vi "DetectCollisionImproved.vi"(0 "ball":dbl[](array[numeric]), 3 "ignoreBall?":bool, 4 "Goal":dbl[](array[numeric]), 5 "our_robots":T1[](array[typedef]), 6 "Initial State":dbl[](array[numeric]), 7 "enemy_robots":T1[](array[typedef]), 8 "Is not first robot?":bool, 9 "element being analyzed":dbl[](array[numeric]), 10 "element already in path":dbl[](array[numeric]), 11 "Robot in":T1={"id"=0, "function"=enum."Attacker", "x"=0.0, "y"=0.0, "orientation"=0.0, "v_tangent"=0.0, "v_normal"=0.0, "v_ang"=0.0, "kick_x"=0.0, "kick_z"=0.0, "dribble"=FALSE, "Timestamp"=timestamp(0 s since 1904-01-01), "estimatives"={"est_v_tangent"=0.0, "est_v_normal"=0.0, "est_vx"=0.0, "est_vy"=0.0, "Pos Robot Est"=[]}, "dest_x_kick"=0.0, "dest_y_kick"=0.0, "Gap Coord"=[], "States"=enum."Pass", "Path "=[], "Path  Smooth"=[], "Dest"=[], "vx_desired"=0.0, "vy_desired"=0.0}) -> (2 "Is there colision?":bool)   [LabVIEW 2018]
uses:
  Vision_class/Old vision/Controls/AI Robot.ctl
  Vision_class/Old vision/Controls/Functions Enum.ctl
  Vision_class/Old vision/Controls/AttackerStates.ctl
  Vision_class/Old vision/Controls/PathDests.ctl
  Vision_class/Old vision/Controls/PathDest.ctl
  <vilib>/Analysis/_algsub.llb/Real Vector Norm.vi
  <vilib>/Analysis/baseanly.llb/Real Dot Product.vi
  <vilib>/Analysis/NI_AALBase.lvlib
  <vilib>/Analysis/NI_AALPro.lvlib
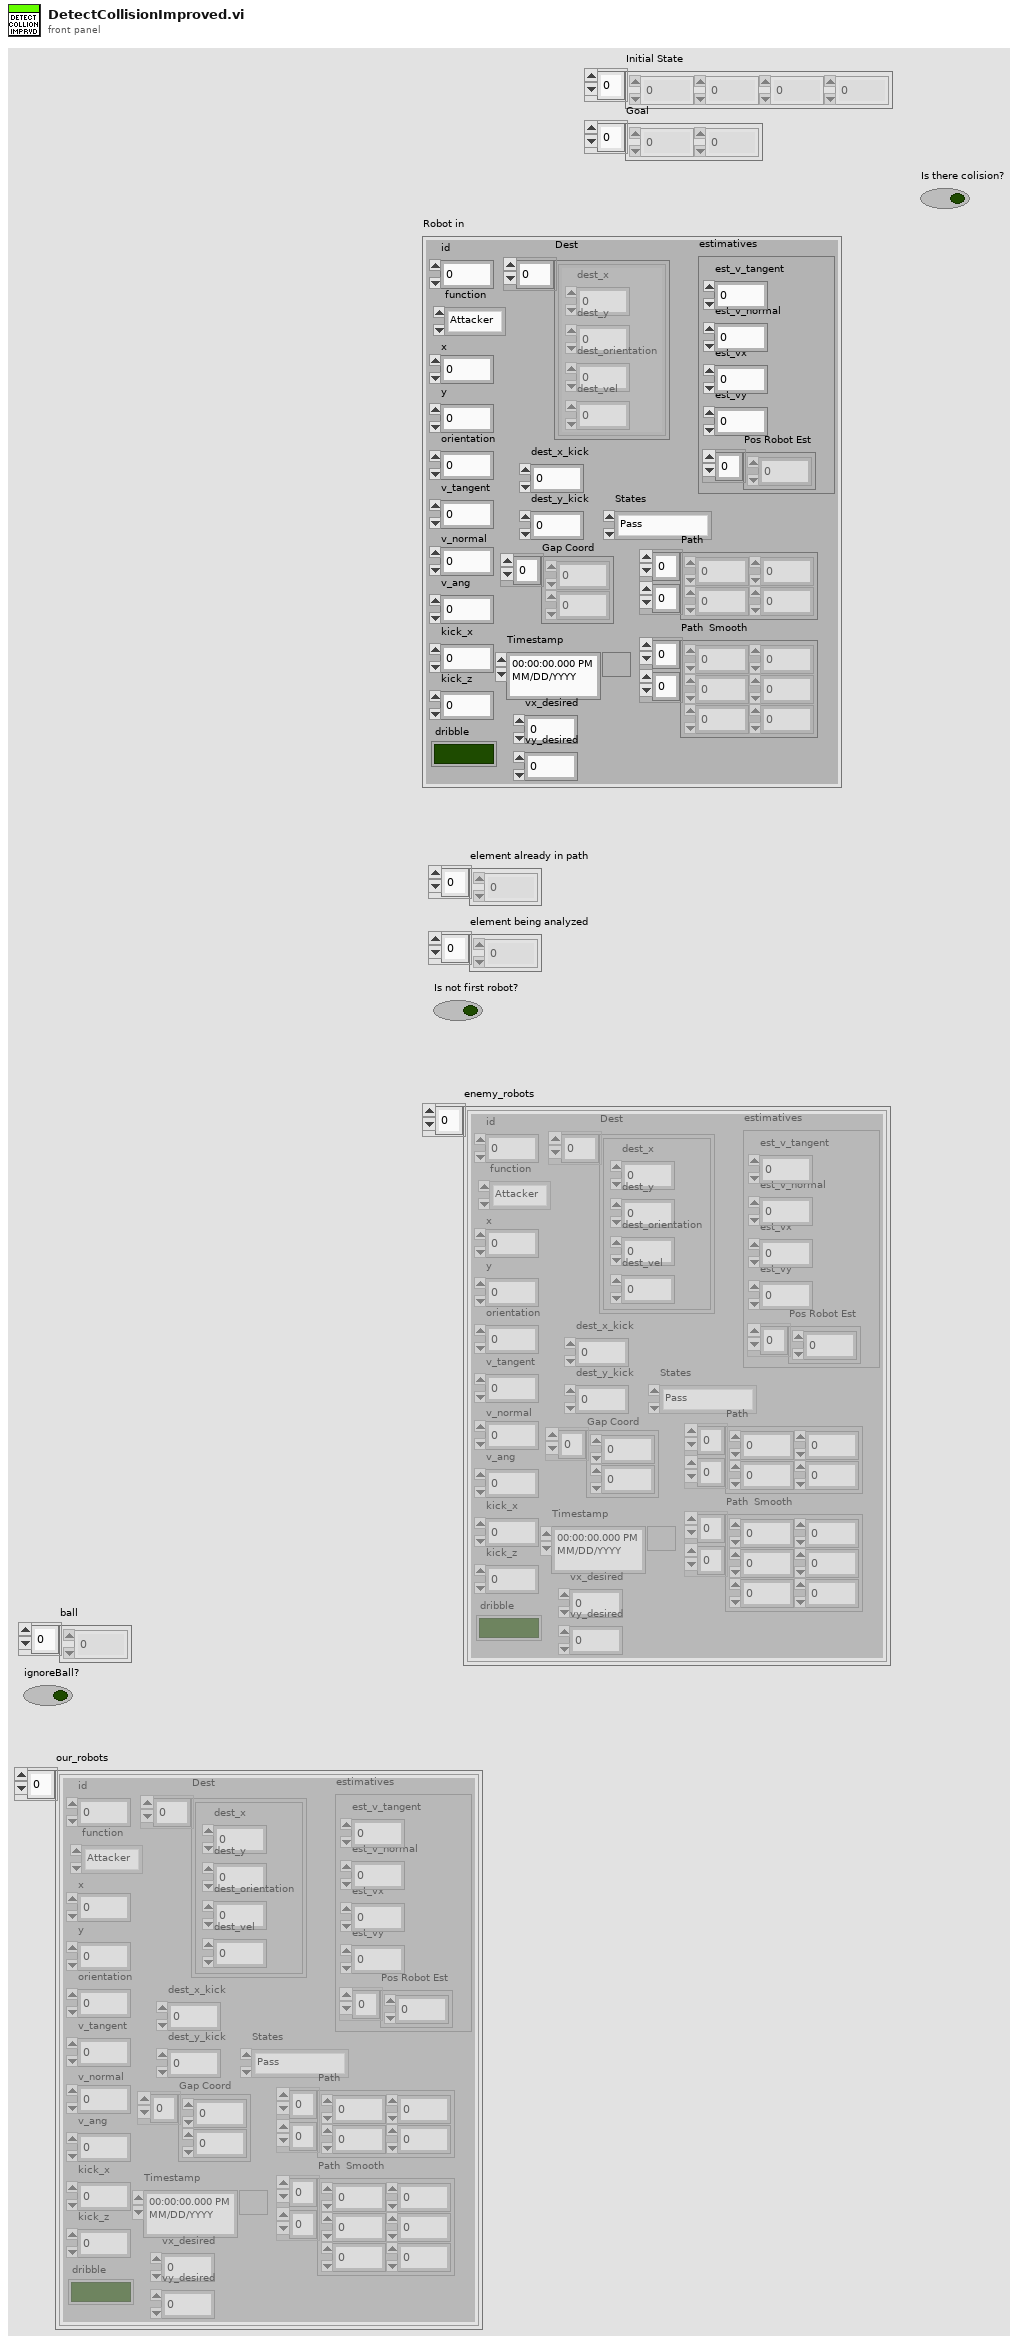
[diagram p1: front panel]
types:
  T1 = typedef "AI Robot.ctl" = cluster{"id":u32, "function":T2, "x":dbl, "y":dbl, "orientation":dbl, "v_tangent":dbl, "v_normal":dbl, "v_ang":dbl, "kick_x":dbl, "kick_z":dbl, "dribble":bool, "Timestamp":timestamp, "estimatives":cluster{"est_v_tangent":dbl, "est_v_normal":dbl, "est_vx":dbl, "est_vy":dbl, "Pos Robot Est":dbl[]}, "dest_x_kick":dbl, "dest_y_kick":dbl, "Gap Coord":dbl[], "States":T3, "Path ":dbl[][], "Path  Smooth":dbl[][], "Dest":T4, "vx_desired":dbl, "vy_desired":dbl}
  T2 = typedef "Functions Enum.ctl" = enum16{"2nd Striker", "Attacker", "Goalie", "Defender", "Striker", "Goto 0", "Dummy", "Kicker", "ZigZag 0", "ZigZag 1", "ZigZag 2", "ZigZag 3", "ZigZag 4", "ZigZag 5", "ZigZag 6", "ZigZag 7", "ZigZag 8", ""}
  T3 = typedef "AttackerStates.ctl" = enum16{"Pass", "GoToTangent", "BallGetting", "GoToKick", ""}
  T4 = typedef "PathDests.ctl" = T5[]
  T5 = typedef "PathDest.ctl" = cluster{"dest_x":dbl, "dest_y":dbl, "dest_orientation":dbl, "dest_vel":dbl}
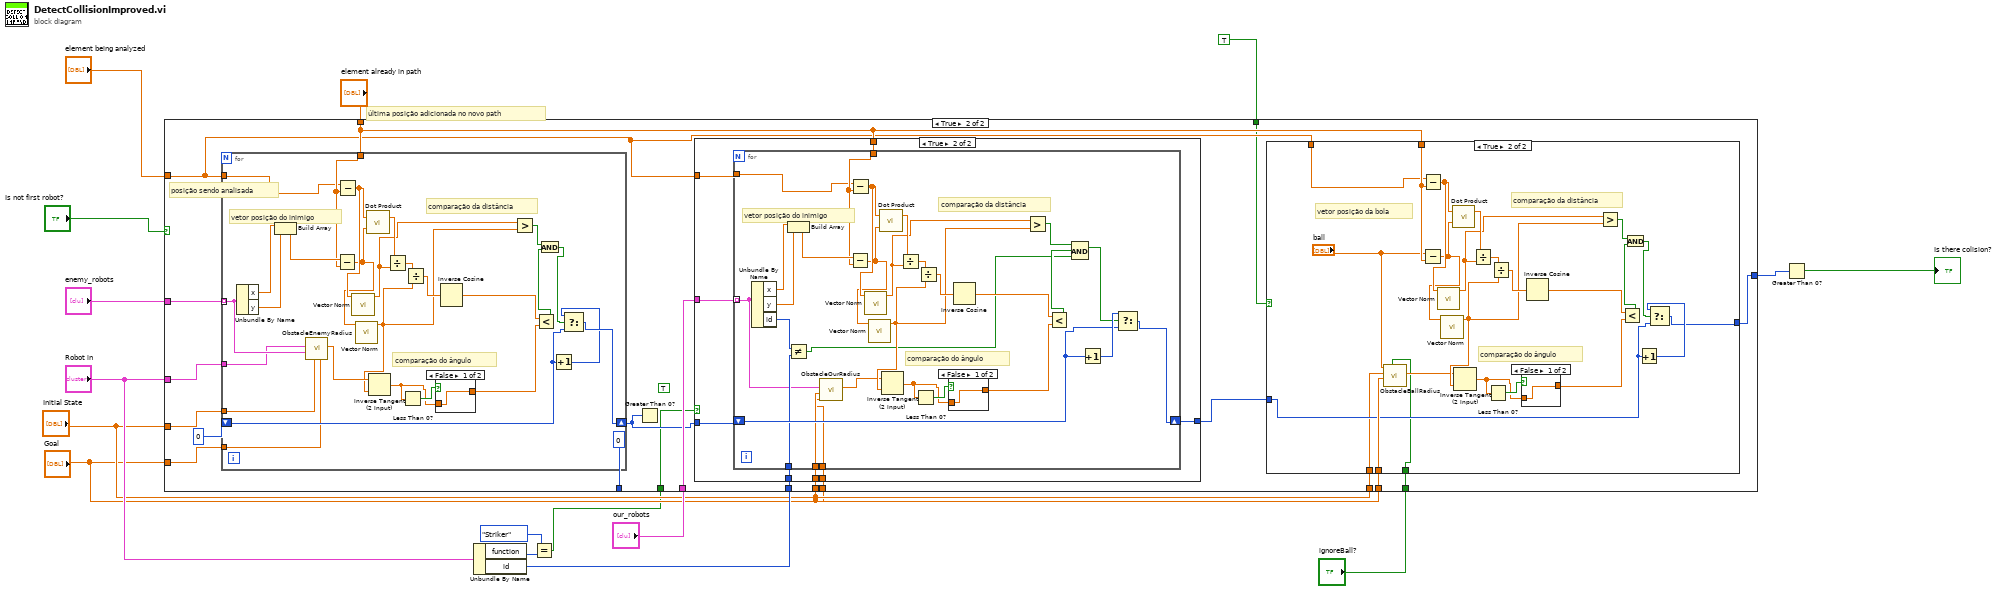
[diagram p0: block diagram]
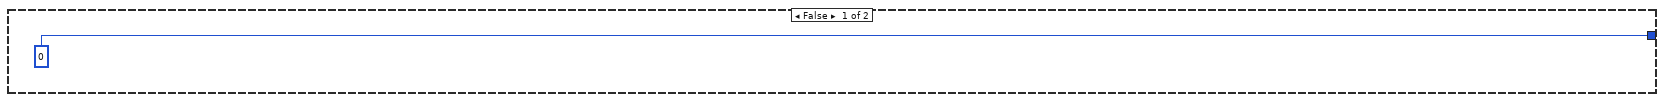
[diagram p2: hidden frame]
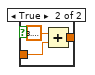
[diagram p4: hidden frame]
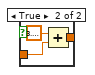
[diagram p6: hidden frame]
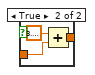
[diagram p7: hidden frame]
diagram:
  # "última posição adicionada no novo path"
  n1 = Unbundle By Name("Robot in") -> ("function"=w4:T2, "id"=w8:u32)
  n2 = Equal?(x=Functions_Enum."Striker", y=w4) -> (x = y?=w2:bool)
  n3 = case shown="True" "Is not first robot?" {
    tunnel: "enemy_robots" -> [_ w37]
    tunnel: "element being analyzed" -> [_ w25]
    tunnel: "element already in path" -> [_ w26]
    tunnel: [0 w22] -> w16
    tunnel: "Robot in" -> [_ w35]
    tunnel: "Initial State" -> [_ w34]
    tunnel: "Goal" -> [_ w33]
    tunnel: 0 -> [_ _]
    tunnel: "our_robots" -> [_ w32]
    tunnel: w8 -> [_ w31]
    tunnel: "Initial State" -> [_ w29]
    tunnel: "Goal" -> [_ w28]
    tunnel: "Initial State" -> [_ w24]
    tunnel: "Goal" -> [_ w23]
    tunnel: TRUE -> [_ w21]
    tunnel: w2 -> [_ w20]
    tunnel: "ignoreBall?" -> [_ w19]
    frame False {
    }
    frame True {
      (unwired) TRUE
      # "posição sendo analisada"
      n4 = for {
        tunnel: w37 -> [w114] mode=indexing
        shift-right: [w124] -> w30
        shift-left: 0 -> [w122]
        tunnel: w25 -> [w131]
        tunnel: w26 -> [w132]
        tunnel: w35 -> [w113]
        tunnel: w34 -> [w112]
        tunnel: w33 -> [w111]
        # "comparação do ângulo"
        # "comparação da distância"
        # "vetor posição do inimigo"
        n5 = Unbundle By Name(w114) -> ("x"=w135:dbl, "y"=w134:dbl)
        n6 = Build Array(w135, w134) -> (w133:dbl[])
        n7 = call "ObstacleEnemyRadius.vi"("Goal"=w111, "Initial State"=w112, "Robot enemy"=w114, "Robot in"=w113) -> ("obstacle enemy radius"=w110:dbl)  [unwired: 7 in]
        n8 = Subtract(x=w133, y=w132) -> (x-y=w125:dbl[])
        n9 = Subtract(x=w131, y=w132) -> (x-y=w129:dbl[])
        n10 = call-poly <vilib>:"Vector Norm.vi"("Input Vector"=w129) -> ("norm"=w121:dbl)  [unwired: 9 in, 1 out]
        n11 = call-poly <vilib>:"Vector Norm.vi"("Input Vector"=w125) -> ("norm"=w109:dbl)  [unwired: 9 in, 1 out]
        n12 = call-poly <vilib>:"Dot Product.vi"("Y Vector"=w125, "X Vector"=w129) -> ("X * Y"=w130:dbl)  [unwired: 1 out]
        n13 = Inverse Tangent (2 Input)(1:w109, 2:w110) -> (0:w116:dbl)
        n14 = Divide(x=w130, y=w121) -> (x/y=w128:dbl)
        n15 = Less Than 0?(x=w116) -> (x < 0?=w117:bool)
        n16 = Divide(x=w128, y=w109) -> (x/y=w127:dbl)
        n17 = case shown="False" w117 {
          tunnel: w116 -> [w136 w138]
          tunnel: [w136 w137] -> w115
          frame False {
          }
          frame True {
            n18 = Add(x=3.141592653589793, y=w138) -> (x+y=w137:dbl)
          }
        }
        n19 = Inverse Cosine(1:w127) -> (0:w126:dbl)
        n20 = Greater?(x=w121, y=w109) -> (0:w120:bool)
        n21 = Less?(x=w126, y=w115) -> (x < y?=w119:bool)
        n22 = And(x=w120, y=w119) -> (x .and. y?=w118:bool)
        n23 = Increment(x=w122) -> (x+1=w123:i32)
        n24 = Select(t=w123, s=w118, f=w122) -> (s? t:f=w124:i32)
      }
      n25 = Greater Than 0?(x=w30) -> ()  [unwired: 1 out]
      n26 = case shown="True" w20 {
        tunnel: w30 -> [w67 w75]
        tunnel: w32 -> [_ w74]
        tunnel: w26 -> [_ w73]
        tunnel: w25 -> [_ w72]
        tunnel: w31 -> [_ w71]
        tunnel: [w67 w70] -> w27
        tunnel: w29 -> [_ w69]
        tunnel: w28 -> [_ w68]
        frame False {
        }
        frame True {
          n27 = for {
            tunnel: w74 -> [w78] mode=indexing
            shift-right: [w93] -> w70
            shift-left: w75 -> [w84]
            tunnel: w72 -> [w100]
            tunnel: w73 -> [w101]
            tunnel: w71 -> [w81]
            tunnel: w69 -> [w77]
            tunnel: w68 -> [w76]
            # "comparação do ângulo"
            # "comparação da distância"
            # "vetor posição do inimigo"
            n28 = Unbundle By Name(w78) -> ("x"=w104:dbl, "y"=w103:dbl, "id"=w82:u32)
            n29 = Build Array(w104, w103) -> (w102:dbl[])
            n30 = Not Equal?(x=w82, y=w81) -> (x != y?=w80:bool)
            n31 = call "ObstacleOurRadius.vi"("Goal"=w76, "Initial State"=w77, "other robot"=w78) -> ("obstacle enemy radius"=w79:dbl)  [unwired: 8 in]
            n32 = Subtract(x=w102, y=w101) -> (x-y=w94:dbl[])
            n33 = Subtract(x=w100, y=w101) -> (x-y=w98:dbl[])
            n34 = call-poly <vilib>:"Vector Norm.vi"("Input Vector"=w98) -> ("norm"=w91:dbl)  [unwired: 9 in, 1 out]
            n35 = call-poly <vilib>:"Vector Norm.vi"("Input Vector"=w94) -> ("norm"=w85:dbl)  [unwired: 9 in, 1 out]
            n36 = call-poly <vilib>:"Dot Product.vi"("Y Vector"=w94, "X Vector"=w98) -> ("X * Y"=w99:dbl)  [unwired: 1 out]
            n37 = Inverse Tangent (2 Input)(1:w85, 2:w79) -> (0:w87:dbl)
            n38 = Divide(x=w99, y=w91) -> (x/y=w97:dbl)
            n39 = Less Than 0?(x=w87) -> (x < 0?=w88:bool)
            n40 = Divide(x=w97, y=w85) -> (x/y=w96:dbl)
            n41 = case shown="False" w88 {
              tunnel: w87 -> [w105 w107]
              tunnel: [w105 w106] -> w86
              frame False {
              }
              frame True {
                n42 = Add(x=3.141592653589793, y=w107) -> (x+y=w106:dbl)
              }
            }
            n43 = Inverse Cosine(1:w96) -> (0:w95:dbl)
            n44 = Greater?(x=w91, y=w85) -> (0:w90:bool)
            n45 = Less?(x=w95, y=w86) -> (x < y?=w89:bool)
            n46 = Compound Arithmetic op=AND(w90, w89, w80) -> (w83:bool)
            n47 = Increment(x=w84) -> (x+1=w92:i32)
            n48 = Select(t=w92, s=w83, f=w84) -> (s? t:f=w93:i32)
          }
        }
      }
      n49 = case shown="True" w21 {
        tunnel: w27 -> [w38 w42]
        tunnel: w26 -> [_ w47]
        tunnel: w25 -> [_ w46]
        tunnel: w24 -> [_ w40]
        tunnel: w23 -> [_ w43]
        tunnel: [w38 w41] -> w22
        tunnel: w19 -> [_ w39]
        frame False {
        }
        frame True {
          # "comparação do ângulo"
          # "comparação da distância"
          # "vetor posição da bola"
          n50 = call "ObstacleBallRadius.vi"("ignoreBall?"=w39, "Goal"=w43, "Initial State"=w40, "ball"="ball") -> ("obstacle enemy radius"=w45:dbl)  [unwired: 7 in]
          n51 = Subtract(x="ball", y=w47) -> (x-y=w57:dbl[])
          n52 = Subtract(x=w46, y=w47) -> (x-y=w61:dbl[])
          n53 = call-poly <vilib>:"Vector Norm.vi"("Input Vector"=w61) -> ("norm"=w55:dbl)  [unwired: 9 in, 1 out]
          n54 = call-poly <vilib>:"Vector Norm.vi"("Input Vector"=w57) -> ("norm"=w48:dbl)  [unwired: 9 in, 1 out]
          n55 = call-poly <vilib>:"Dot Product.vi"("Y Vector"=w57, "X Vector"=w61) -> ("X * Y"=w62:dbl)  [unwired: 1 out]
          n56 = Inverse Tangent (2 Input)(1:w48, 2:w45) -> (0:w50:dbl)
          n57 = Divide(x=w62, y=w55) -> (x/y=w60:dbl)
          n58 = Less Than 0?(x=w50) -> (x < 0?=w51:bool)
          n59 = Divide(x=w60, y=w48) -> (x/y=w59:dbl)
          n60 = case shown="False" w51 {
            tunnel: w50 -> [w63 w65]
            tunnel: [w63 w64] -> w49
            frame False {
            }
            frame True {
              n61 = Add(x=3.141592653589793, y=w65) -> (x+y=w64:dbl)
            }
          }
          n62 = Inverse Cosine(1:w59) -> (0:w58:dbl)
          n63 = Greater?(x=w55, y=w48) -> (0:w54:bool)
          n64 = Less?(x=w58, y=w49) -> (x < y?=w53:bool)
          n65 = And(x=w54, y=w53) -> (x .and. y?=w52:bool)
          n66 = Increment(x=w42) -> (x+1=w56:i32)
          n67 = Select(t=w56, s=w52, f=w42) -> (s? t:f=w41:i32)
        }
      }
    }
  }
  n68 = Greater Than 0?(x=w16) -> (x > 0?=→"Is there colision?":bool)
